vi "SEA_9811_Init.vi"(7 "Run?":bool=TRUE, 8 "error in":errorcluster, 9 "Transmit Channels Ref in":T1 format="%.0x", 10 "SEA9811_conf_cluster":T9={"FPGA resource name"="RIO0", "Rx ch conf (0..7)"=[{"Rx Channel Number (0..7)"=0, "Rx Label Filter"={"Label 00"=0, "Label 01"=0, "Label 02"=0, "Label 03"=0, "Label 04"=0, "Label 05"=0, "Label 06"=0, "Label 07"=0, "Label 08"=0, "Label 09"=0, "Label 10"=0, "Label 11"=0, "Label 12"=0, "Label 13"=0, "Label 14"=0, "Label 15"=0}, "Receiver Control Register (RCR)"={"RCR0: Data rate = ARINC 429 High-Speed (0) or Low-Speed (1)"=FALSE, "RCR1: not used"=FALSE, "RCR2: Label recognition for this channel enabled (1) or disabled (0)"=FALSE, "RCR3: Receiver channel disabled (1) or enabled (0)"=FALSE, "RCR4: Odd parity check for this channel enabled (1) or disabled (0"=FALSE, "RCR5: Receiver normal operation (1) or loopback mode (0)"=TRUE, "RCR6: Receiver Decoder disabled (0) or enabled (1) \n-> ARINC bits 10 and 9 must match RCR7 and RCR8"=FALSE, "RCR7: If receiver decoder is enabled (RCR6=1), \nthe ARINC bit 10 must match this bit"=FALSE, "RCR8: If receiver decoder is enabled (RCR6=1), \nthe ARINC bit 9 must match this bit"=FALSE, "RCR9: Label bit order for this channel non-reversed (1) \nor reversed (0)"=FALSE, "RCR10: not used"=FALSE, "RCR11: not used"=FALSE, "RCR12: not used"=FALSE, "RCR13: not used"=FALSE, "RCR14: not used"=FALSE, "RCR15: not used"=FALSE}}], "Transmitter Control Register (TCR)"={"TCR0: not used"=FALSE, "TCR1: not used"=FALSE, "TCR2: not used"=FALSE, "TCR3: Transmitter Parity Bit Enable: 32nd bit is parity (1) or data (0)"=FALSE, "TCR4: not used"=FALSE, "TCR5: not used"=FALSE, "TCR6: not used"=FALSE, "TCR7: not used"=FALSE, "TCR8: not used"=FALSE, "TCR9: Transmitter Parity Select: odd parity (0) or even parity (1)"=FALSE, "TCR10: Transmitter Data Rate: ARINC 429 high-speed (0) or low-speed (1)"=FALSE, "TCR11: ARINC Label Bit Order: label bit order reversed (0) or not reversed (1)"=FALSE, "TCR12: Disable Line Driver: normal operation (0) or transmitter disabled (1)"=FALSE, "TCR13: Tansmit whenever data is available in FIFO (1) or only start by instruction \"Enable Transmission\" (0)"=TRUE, "TCR14: not used"=FALSE, "TCR15: not used"=FALSE}, "Bitfile Path"=path ""}, 11 "Device Reference in":T1 format="%.0x") -> (0 "error out":errorcluster, 2 "SEA9811_RT_data out":T2 {"Tx"."Tx Refs (Data,Trig)"."Data Reference" format="%.0x"}, 3 "Device Reference out":T1 format="%.0x")   [LabVIEW 2012]
uses:
  Typdefs/SEA9811_RT_conf_cluster.ctl
  <vilib>/userdefined/High Color/nirio_resource_hc.ctl
  FPGA/SEA-9811_ReceiverAndTransmitter/SubVIs/SEA-9811_ReceiverAndTransmitter_RCR.ctl
  FPGA/SEA-9811_ReceiverAndTransmitter/SubVIs/SEA-9811_ReceiverAndTransmitter_TCR.ctl
  Typdefs/SEA9811_RT_data_cluster.ctl
  <userlib>/_FPGA Interface Advanced Tools/FPGA Interface Base/FPGA Interface Base.lvclass
  Typdefs/FPGA ref.ctl
  Typdefs/channel.ctl
  Typdefs/received word.ctl
  Typdefs/SEA9811_FPGA_FP_Addresses.ctl
  <vilib>/NI Veristand/Custom Device API/Block Data Reference.ctl
  <vilib>/NI Veristand/Custom Device API/Data Reference.ctl
  <vilib>/NI Veristand/Custom Device API/Custom Device Item Ref.ctl
  <vilib>/NI Veristand/Custom Device API/Data Access Type.ctl
  <vilib>/NI Veristand/Custom Device API/Custom Device API.lvlib
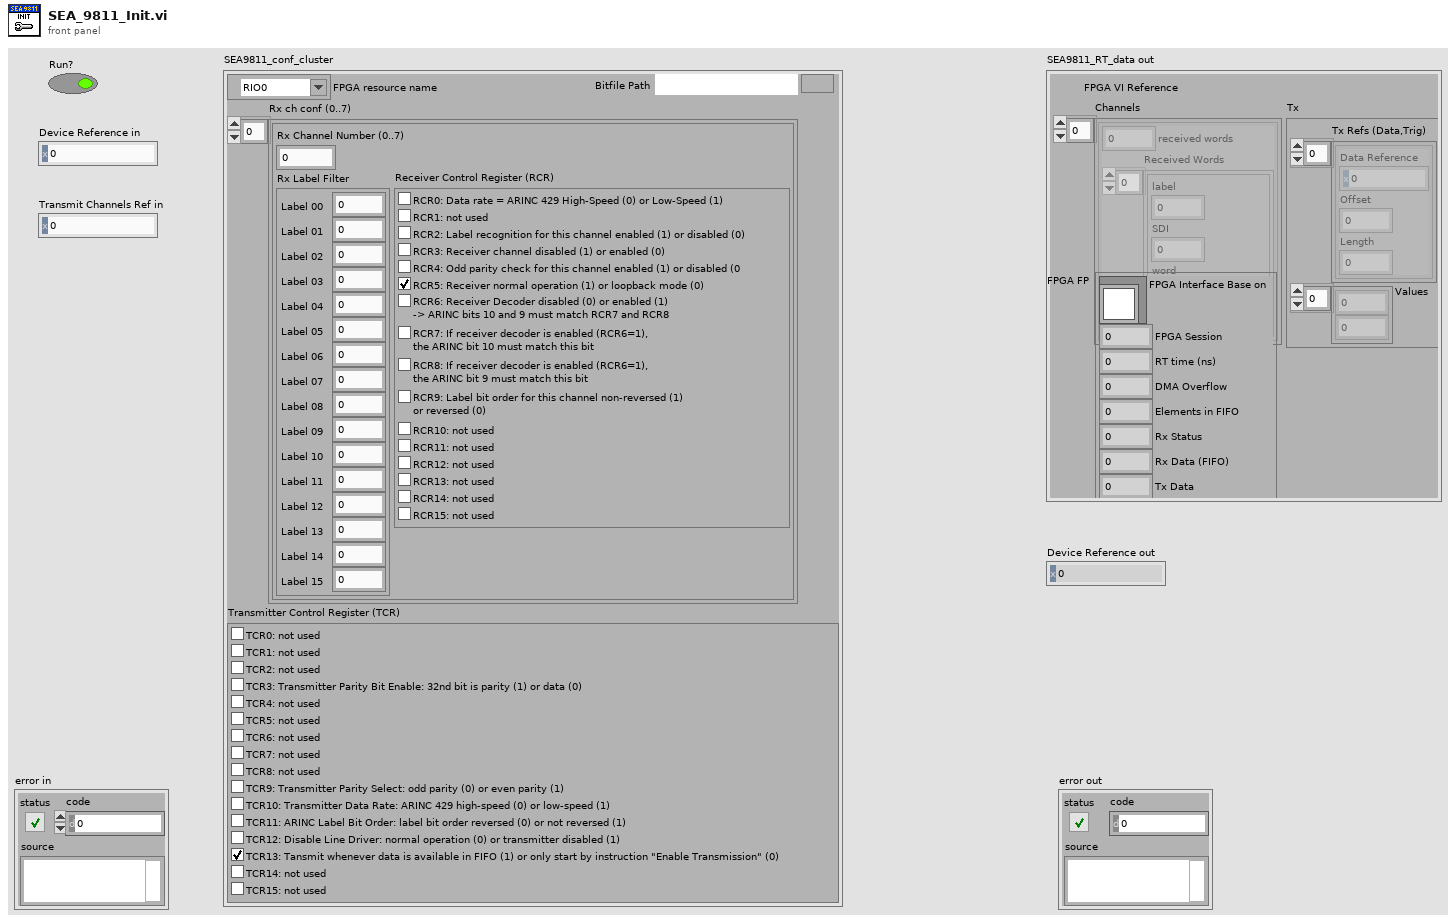
[diagram p1: front panel]
types:
  T1 = typedef "Custom Device API.lvlib/Custom Device Item Ref.ctl" = u64
  T2 = typedef "SEA9811_RT_data_cluster.ctl" = cluster{"FPGA VI Reference":T3, "Channels":T4[], "FPGA FP":T6, "Tx":cluster{"Tx Refs (Data,Trig)":T7[], "Values":dbl[]}}
  T3 = typedef "FPGA ref.ctl" = refnum<k20>
  T4 = typedef "channel.ctl" = cluster{"received words":u32, "Received Words":T5[]}
  T5 = typedef "received word.ctl" = cluster{"label":u8, "SDI":u8, "word":u32, "timestamp":dbl}
  T6 = typedef "SEA9811_FPGA_FP_Addresses.ctl" = cluster{"FPGA Interface Base on":refnum<class "FPGA Interface Base.lvclass">, "FPGA Session":u32, "RT time (ns)":u32, "DMA Overflow":u32, "Elements in FIFO":u32, "Rx Status":u32, "Rx Data (FIFO)":u32, "Tx Data":u32, "Transmit Data":u32}
  T7 = typedef "Custom Device API.lvlib/Block Data Reference.ctl" = cluster{"Data Reference":T8, "Offset":i32, "Length":i32}
  T8 = typedef "Custom Device API.lvlib/Data Reference.ctl" = i32
  T9 = typedef "SEA9811_RT_conf_cluster.ctl" = cluster{"FPGA resource name":T10, "Rx ch conf (0..7)":cluster{"Rx Channel Number (0..7)":u8, "Rx Label Filter":cluster{"Label 00":u8, "Label 01":u8, "Label 02":u8, "Label 03":u8, "Label 04":u8, "Label 05":u8, "Label 06":u8, "Label 07":u8, "Label 08":u8, "Label 09":u8, "Label 10":u8, "Label 11":u8, "Label 12":u8, "Label 13":u8, "Label 14":u8, "Label 15":u8}, "Receiver Control Register (RCR)":T11}[], "Transmitter Control Register (TCR)":T12, "Bitfile Path":path}
  T10 = typedef "nirio_resource_hc.ctl" = tag
  T11 = typedef "SEA-9811_ReceiverAndTransmitter_RCR.ctl" = cluster{"RCR0: Data rate = ARINC 429 High-Speed (0) or Low-Speed (1)":bool, "RCR1: not used":bool, "RCR2: Label recognition for this channel enabled (1) or disabled (0)":bool, "RCR3: Receiver channel disabled (1) or enabled (0)":bool, "RCR4: Odd parity check for this channel enabled (1) or disabled (0":bool, "RCR5: Receiver normal operation (1) or loopback mode (0)":bool, "RCR6: Receiver Decoder disabled (0) or enabled (1) \n-> ARINC bits 10 and 9 must match RCR7 and RCR8":bool, "RCR7: If receiver decoder is enabled (RCR6=1), \nthe ARINC bit 10 must match this bit":bool, "RCR8: If receiver decoder is enabled (RCR6=1), \nthe ARINC bit 9 must match this bit":bool, "RCR9: Label bit order for this channel non-reversed (1) \nor reversed (0)":bool, "RCR10: not used":bool, "RCR11: not used":bool, "RCR12: not used":bool, "RCR13: not used":bool, "RCR14: not used":bool, "RCR15: not used":bool}
  T12 = typedef "SEA-9811_ReceiverAndTransmitter_TCR.ctl" = cluster{"TCR0: not used":bool, "TCR1: not used":bool, "TCR2: not used":bool, "TCR3: Transmitter Parity Bit Enable: 32nd bit is parity (1) or data (0)":bool, "TCR4: not used":bool, "TCR5: not used":bool, "TCR6: not used":bool, "TCR7: not used":bool, "TCR8: not used":bool, "TCR9: Transmitter Parity Select: odd parity (0) or even parity (1)":bool, "TCR10: Transmitter Data Rate: ARINC 429 high-speed (0) or low-speed (1)":bool, "TCR11: ARINC Label Bit Order: label bit order reversed (0) or not reversed (1)":bool, "TCR12: Disable Line Driver: normal operation (0) or transmitter disabled (1)":bool, "TCR13: Tansmit whenever data is available in FIFO (1) or only start by instruction \"Enable Transmission\" (0)":bool, "TCR14: not used":bool, "TCR15: not used":bool}
  T13 = typedef "Custom Device API.lvlib/Data Access Type.ctl" = enum16{"Read", "Write"}
  T14 = cluster{"Rx Channel Number (0..7)":u8, "Rx Label Filter":cluster{"Label 00":u8, "Label 01":u8, "Label 02":u8, "Label 03":u8, "Label 04":u8, "Label 05":u8, "Label 06":u8, "Label 07":u8, "Label 08":u8, "Label 09":u8, "Label 10":u8, "Label 11":u8, "Label 12":u8, "Label 13":u8, "Label 14":u8, "Label 15":u8}, "Receiver Control Register (RCR)":T11}[]
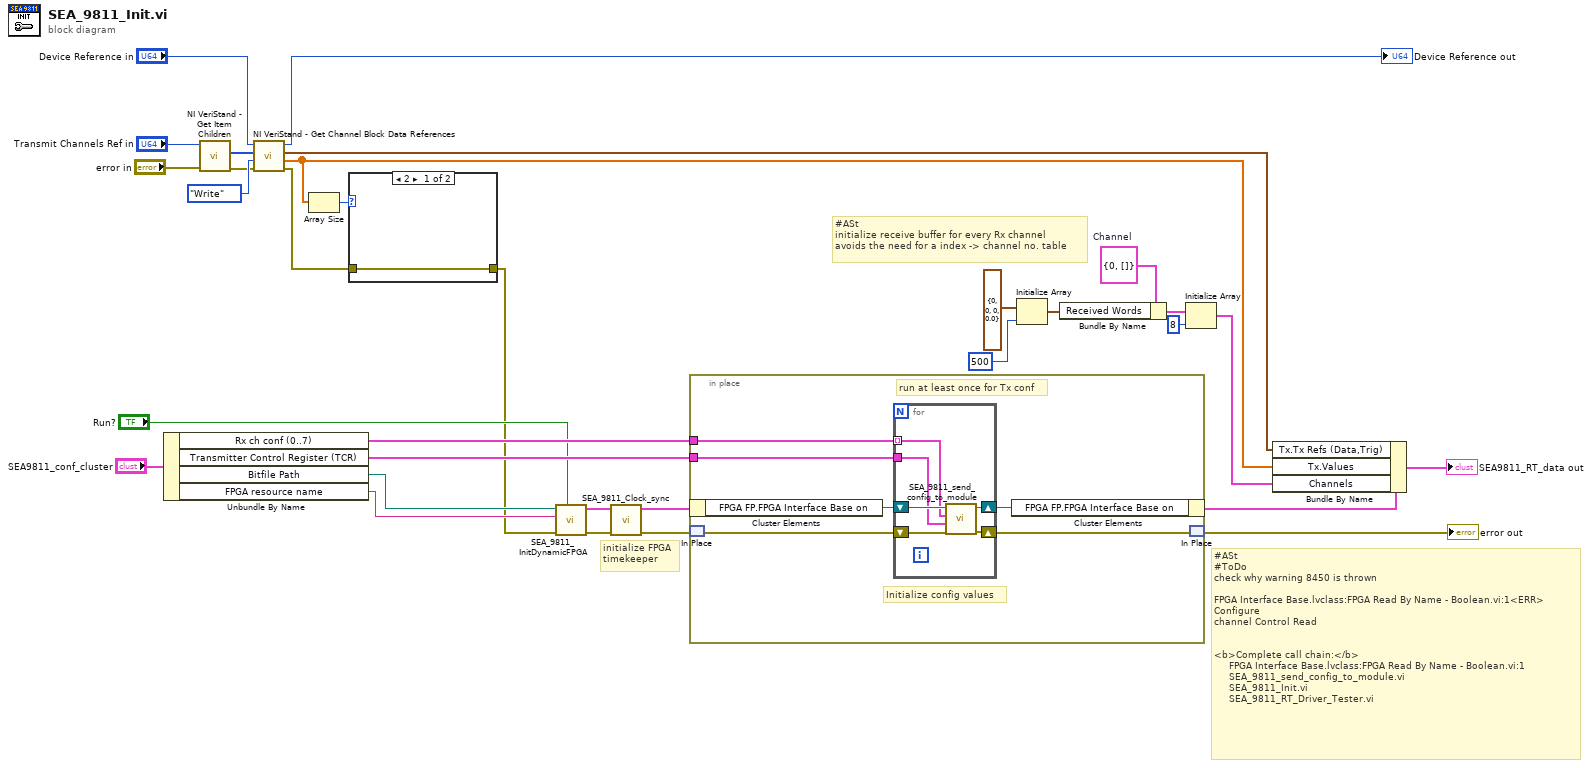
[diagram p0: block diagram]
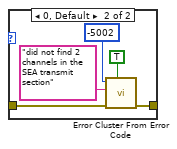
[diagram p2: hidden frame]
diagram:
  w26 = T4 {"received words"=0, "Received Words"=[]}  # Channel
  # "#ASt\n#ToDo\ncheck why warning 8450 is thrown\n\nFPGA Interface Base.lvclass:FPGA Read By Name - Boolean.vi:1<ERR>\nConfigure\nchannel Control Read\n\n\n<b>Complete call chain:</b>\n     FPGA Interface Base.lvclass:FPGA Read By Name - Boolean.vi:1\n     SEA_9811_send_config_to_module.vi\n     SEA_9811_Init.vi\n     SEA_9811_RT_Driver_Tester.vi"
  # "initialize FPGA\ntimekeeper"
  # "#ASt \ninitialize receive buffer for every Rx channel\navoids the need for a index -> channel no. table"
  n1 = Unbundle By Name("SEA9811_conf_cluster") -> ("Rx ch conf (0..7)"=w31:T14, "Transmitter Control Register (TCR)"=w30:T12, "Bitfile Path"=w20:path, "FPGA resource name"=w21:T10)
  n2 = call <vilib>:"NI VeriStand - Get Item Children.vi"("error in (no error)"="error in", "Item Ref in"="Transmit Channels Ref in") -> ("error out"=w7:errorcluster, "Child Refs"=w11:T1[])  [unwired: 6 in, 2 out]
  n3 = call <vilib>:"NI VeriStand - Get Channel Block Data References.vi"("error in (no error)"=w7, "Access"=Data_Access_Type."Write", "Channel Refs"=w11, "Device Ref in"="Device Reference in") -> ("error out"=w5:errorcluster, "Values Array"=w2:dbl[], "Block Data Refs"=w1:T7[], "Device Ref out"=→"Device Reference out":T1)  [unwired: 4 in]
  n4 = Array Size(array=w2) -> (size(s)=w6:i32)
  n5 = case shown="2" w6 {
    tunnel: w5 -> [w33 w36]
    tunnel: [w33 w35] -> w3
    frame 2 {
    }
    frame 0, Default {
      n6 = call <vilib>:"Error Cluster From Error Code.vi"("show call chain? (False)"=TRUE, "error in (no error)"=w36, "error message (\"\")"="did not find 2 channels in the SEA transmit section" ("error message (\"\")"), "error code (0)"=-5002) -> ("error out"=w35:errorcluster)  [unwired: 5 in]
    }
  }
  n7 = call "SEA_9811_InitDynamicFPGA.vi"("Run?"="Run?", "error in (no error)"=w3, "FPGA resource name"=w21, "Bitfile Path"=w20) -> ("error out"=w14:errorcluster, "SEA9811_RT_data out"=w16:T2)  [unwired: 6 in]
  n8 = call "SEA_9811_Clock_sync.vi"("error in (no error)"=w14, "SEA9811_RT_data in"=w16) -> ("error out"=w13:errorcluster, "SEA9811_RT_data out"=w15:T2)  [unwired: 8 in]
  n9 = in-place {
    in-place-border: w31 -> [w44]
    in-place-border: w30 -> [w43]
    # "run at least once for Tx conf"
    # "Initialize config values"
    n10 = in-place-cluster #1(w15) -> ("FPGA FP.FPGA Interface Base on"=w40:refnum<class "FPGA Interface Base.lvclass">)
    n11 = in-place-match #2(w13) -> (w41:errorcluster)
    n12 = for {
      shift-right: [w47] -> w42
      shift-left: w41 -> [w49]
      shift-right: [w48] -> w39
      shift-left: w40 -> [w50]
      tunnel: w44 -> [w46] mode=indexing
      tunnel: w43 -> [w45]
      n13 = call "SEA_9811_send_config_to_module.vi"("error in (no error)"=w49, "Transmitter Control Register (TCR)"=w45, "Rx channel"=w46, "FPGA Interface Base In"=w50) -> ("error out"=w47:errorcluster, "FPGA Interface Base Out"=w48:refnum<class "FPGA Interface Base.lvclass">)  [unwired: 6 in]
    }
    n14 = in-place-cluster #1("FPGA FP.FPGA Interface Base on"=w39) -> (w17:T2)
    n15 = in-place-match #2(w42) -> (→"error out":errorcluster)
  }
  n16 = Initialize Array(T5 {"label"=0, "SDI"=0, "word"=0, "timestamp"=0.0} ("received word"), 500 ("dimension size")) -> (w25:T5[])
  n17 = Bundle By Name(cluster=w26, "Received Words"=w25) -> (w24:T4)
  n18 = Initialize Array(w24, 8 ("dimension size")) -> (w22:T4[])
  n19 = Bundle By Name(cluster=w17, "Tx.Tx Refs (Data,Trig)"=w1, "Tx.Values"=w2, "Channels"=w22) -> (→"SEA9811_RT_data out":T2)
